vi "Datas to Plot.vi"(4 "Ellipse Length":dbl[](array[numeric]), 6 "Motor Configuration":dbl[][](array[numeric]), 7 "Reference Position":dbl[](array[numeric]), 8 "Shfted Reference":dbl[](array[numeric]), 9 "Cable Length":dbl[](array[numeric]), 10 "Arrow":dbl[](array[numeric]), 11 "Measured Position":dbl[](array[numeric])) -> (3 "Plot":cluster{dbl[], dbl[]}[](array[cluster]))   [LabVIEW 2021]
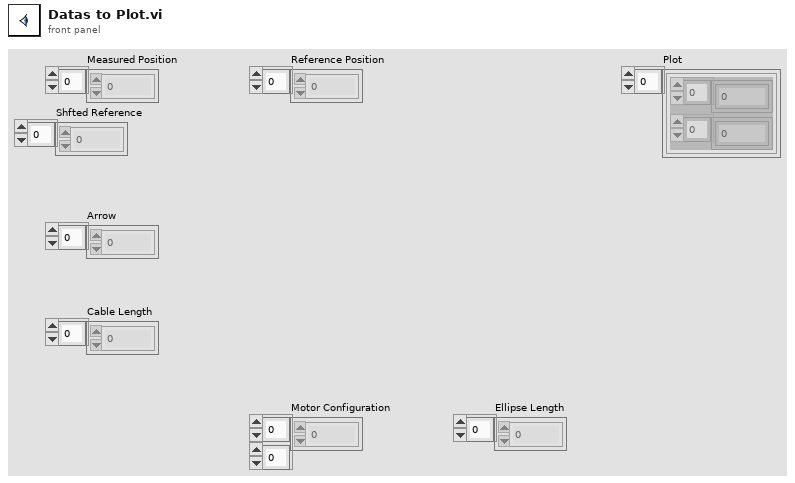
[diagram p1: front panel]
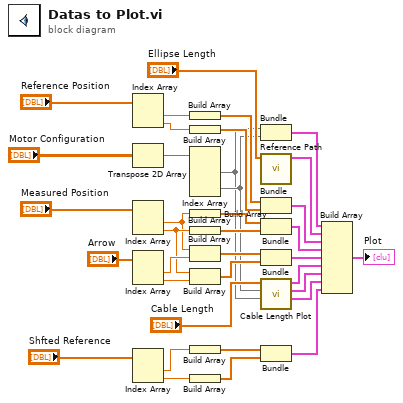
[diagram p0: block diagram]
diagram:
  n1 = Index Array(array="Reference Position") -> (element #1=w28:dbl, element #2=w27:dbl)  [unwired: 2 in]
  n2 = Transpose 2D Array(2D array="Motor Configuration") -> (transposed array=w26:dbl[][])
  n3 = Index Array(array="Measured Position") -> (element #1=w31:dbl, element #2=w32:dbl)  [unwired: 2 in]
  n4 = Index Array(array="Arrow") -> (element #1=w35:dbl, element #2=w36:dbl)  [unwired: 2 in]
  n5 = Index Array(array="Shfted Reference") -> (element #1=w3:dbl, element #2=w2:dbl)  [unwired: 2 in]
  n6 = Build Array(w28) -> (w24:dbl[])
  n7 = Build Array(w27) -> (w25:dbl[])
  n8 = Index Array(array=w26) -> (element #1=w17:dbl[], element #2=w18:dbl[])  [unwired: 4 in]
  n9 = Build Array(w31) -> (w29:dbl[])
  n10 = Build Array(w32) -> (w30:dbl[])
  n11 = Build Array(w31, w35) -> (w33:dbl[])
  n12 = Build Array(w32, w36) -> (w34:dbl[])
  n13 = Build Array(w3) -> (w6:dbl[])
  n14 = Build Array(w2) -> (w5:dbl[])
  n15 = Bundle(w17, w18) -> (w9:cluster{dbl[], dbl[]})  [unwired: 1 in]
  n16 = call "Reference Path.vi"("a,b"="Ellipse Length") -> ("Circular Path"=w10:cluster{dbl[], dbl[]})  [unwired: 10 in]
  n17 = Bundle(w24, w25) -> (w11:cluster{dbl[], dbl[]})  [unwired: 1 in]
  n18 = Bundle(w29, w30) -> (w12:cluster{dbl[], dbl[]})  [unwired: 1 in]
  n19 = Bundle(w33, w34) -> (w13:cluster{dbl[], dbl[]})  [unwired: 1 in]
  n20 = call "Cable Length Plot.vi"("Motor Config X"=w17, "Motor Config Y"=w18, "Cable Length"="Cable Length") -> ("Circle 3"=w21:cluster{dbl[], dbl[]}, "Circle 2"=w20:cluster{dbl[], dbl[]}, "Circle 1"=w19:cluster{dbl[], dbl[]})  [unwired: 6 in]
  n21 = Bundle(w6, w5) -> (w4:cluster{dbl[], dbl[]})  [unwired: 1 in]
  n22 = Build Array(w9, w10, w11, w12, w13, w19, w20, w21, w4) -> (→"Plot":cluster{dbl[], dbl[]}[])
